vi "Begin.vi"() -> (0 "error out":errorcluster)   [LabVIEW 2013]
doc: "Called before other user functions, this VI is expected to open initial I/O refnums, load in file data, and do all program initialization. Notice that the <B>error out</B> terminal is simply used for data flow. Wiring it to other structures or subVIs ensures that this VI runs first."
uses:
  <vilib>/Rock Robotics/WPI/DriverStation/WPI_DriverStationRobotMode2.ctl
  <vilib>/Rock Robotics/WPI/Joystick/WPI_JoystickDeviceEnum.ctl
  <vilib>/Rock Robotics/SystemInterfaces/DIO/FPGA_DIOPWMChannel.ctl
  <vilib>/Rock Robotics/SystemInterfaces/Typedef/FPGA_TypedefDigitalModule.ctl
  <vilib>/Rock Robotics/SystemInterfaces/DIO/FPGA_DIOChannel.ctl
  <vilib>/Rock Robotics/SystemInterfaces/Typedef/FPGA_TypedefAnalogModuleForGyro.ctl
  <vilib>/Rock Robotics/SystemInterfaces/AI/FPGA_AIGyroChannel.ctl
  <vilib>/Rock Robotics/WPI/Solenoid/WPI_SolenoidChannel.ctl
  <vilib>/Rock Robotics/SystemInterfaces/AI/FPGA_AIChannel.ctl
  <vilib>/Rock Robotics/SystemInterfaces/DIO/FPGA_DIORelayChannel.ctl
  <vilib>/Rock Robotics/WPI/Relay/WPI_RelayDirection.ctl
  <vilib>/Rock Robotics/SystemInterfaces/Typedef/FPGA_TypedefSolenoidModule.ctl
  <vilib>/Rock Robotics/WPI/Solenoid/WPI_SolenoidValue.ctl
  <vilib>/Rock Robotics/WPI/SafetyOutput/WPI_SafetyOutputConfigMenu.ctl
  Robot Global Data.vi
  <vilib>/Rock Robotics/WPI/MotorControl/WPI_MotorControlOpen Talon.vi
  <vilib>/Rock Robotics/WPI/Counter/WPI_CounterDigitalInputToDigitalSource.vi
  <vilib>/Rock Robotics/WPI/Counter/WPI_CounterOpen Semi Period Mode.vi
  <vilib>/Rock Robotics/WPI/Solenoid/WPI_SolenoidOpenSingle.vi
  <vilib>/Rock Robotics/WPI/Solenoid/WPI_SolenoidOpenDouble.vi
  <vilib>/Rock Robotics/WPI/Solenoid/WPI_SolenoidSetEnum.vi
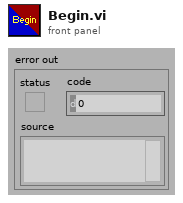
[diagram p1: front panel]
types:
  T1 = typedef "WPI_SafetyOutputConfigMenu.ctl" = enum16{"Enable", "Disable"}
  T2 = typedef "WPI_SolenoidValue.ctl" = enum16{"Off", "On", "Forward", "Reverse"}
  T3 = typedef "FPGA_AIChannel.ctl" = enum8{"AI 1", "AI 2", "AI 3", "AI 4", "AI 5", "AI 6", "AI 7", "AI 8", "Invalid"}
  T4 = typedef "WPI_SolenoidChannel.ctl" = enum8{"Solenoid 1", "Solenoid 2", "Solenoid 3", "Solenoid 4", "Solenoid 5", "Solenoid 6", "Solenoid 7", "Solenoid 8", "Invalid"}
  T5 = typedef "FPGA_TypedefSolenoidModule.ctl" = enum16{"Solenoid Module 1", "Solenoid Module 2"}
  T6 = typedef "WPI_RelayDirection.ctl" = enum16{"Both directions", "Forward only", "Reverse only"}
  T7 = typedef "FPGA_DIORelayChannel.ctl" = enum8{"Relay 1", "Relay 2", "Relay 3", "Relay 4", "Relay 5", "Relay 6", "Relay 7", "Relay 8", "Invalid"}
  T8 = typedef "FPGA_DIOPWMChannel.ctl" = enum8{"PWM 1", "PWM 2", "PWM 3", "PWM 4", "PWM 5", "PWM 6", "PWM 7", "PWM 8", "PWM 9", "PWM 10", "Invalid"}
  T9 = typedef "FPGA_TypedefDigitalModule.ctl" = enum16{"Digital Module 1", "Digital Module 2"}
  T10 = typedef "FPGA_DIOChannel.ctl" = enum8{"DIO 1", "DIO 2", "DIO 3", "DIO 4", "DIO 5", "DIO 6", "DIO 7", "DIO 8", "DIO 9", "DIO 10", "DIO 11", "DIO 12", "DIO 13", "DIO 14", "Invalid"}
  T11 = typedef "WPI_JoystickDeviceEnum.ctl" = enum16{"USB 1", "USB 2", "USB 3", "USB 4", "Kinect 1", "Kinect 2"}
  T12 = typedef "FPGA_AIGyroChannel.ctl" = enum8{"AI 1", "AI 2", "Invalid"}
  T13 = typedef "FPGA_TypedefAnalogModuleForGyro.ctl" = enum16{"Analog Module 1"}
  T14 = typedef "WPI_DriverStationRobotMode2.ctl" = enum16{"Autonomous Disabled", "Autonomous Enabled", "Teleop Disabled", "Teleop Enabled", "Timeout", "Finish", "Test Disabled", "Test Enabled"}
  T15 = typedef "WPI_SolenoidDevRef.ctl" = cluster{"DevStatus":errorcluster, "Solenoid Module":T5, "Forward Solenoid Channel":T4, "Reverse Solenoid Channel":T4}
  T16 = typedef "WPI_JoystickDevRef.ctl" = cluster{"Device":T11}
  T17 = typedef "WPI_AnalogChannelDevRef.ctl" = cluster{"DevStatus":errorcluster, "Analog Module":T18, "Analog Channel":T3}
  T18 = typedef "FPGA_TypedefAnalogModule.ctl" = enum16{"Analog Module 1", "Analog Module 2"}
  T19 = typedef "WPI_DigitalInputDevRef.ctl" = cluster{"DevStatus":errorcluster, "DIO Channel":T10, "Digital Module":T9}
  T20 = typedef "WPI_ServoDeviceRef.ctl" = cluster{"DeviceStatus":errorcluster, "Digital Module":T9, "PWM Channel":T8, "DeadBand":T21}
  T21 = typedef "WPI_PWMDeadband.ctl" = cluster{"Name":string, "maxPositivePwm":i32, "minPositivePwm":i32, "centerPwm":i32, "maxNegativePwm":i32, "minNegativePwm":i32, "angularRange":u16}
  T22 = typedef "FPGA_CounterEncoderSourceConvertionLVSourceType.ctl" = cluster{"DevStatus":errorcluster, "AnalogTriggerMode?":bool, "DigitalMode":cluster{"Digital Module":T9, "DIO Channel":T23}, "AnalogTriggerMode":cluster{"AnalogTriggerIndex":T24, "OutputType":T25}}
  T23 = typedef "FPGA_DIODigitalSourceChannel.ctl" = enum8{"DIO 1", "DIO 2", "DIO 3", "DIO 4", "DIO 5", "DIO 6", "DIO 7", "DIO 8", "DIO 9", "DIO 10", "DIO 11", "DIO 12", "DIO 13", "DIO 14", "Disabled"}
  T24 = typedef "FPGA_AnalogTriggerIndex.ctl" = enum8{"Trig 0", "Trig 1", "Trig 2", "Trig 3", "Trig 4", "Trig 5", "Trig 6", "Trig 7", "Invalid"}
  T25 = typedef "FPGA_AnalogTriggerOutType.ctl" = enum16{"InWindow", "TriggerState", "Rising", "Falling"}
  T26 = typedef "WPI_RelayDevRef.ctl" = cluster{"DevStatus":errorcluster, "Relay Channel":T7, "Digital Module":T9, "Relay Direction":T6}
  T27 = typedef "WPI_MotorControlDeviceRef.ctl" = cluster{"DeviceStatus":errorcluster, "Type":enum16{"PWM", "CAN"}, "PWM":cluster{"Digital Module":T9, "PWM Channel":T8, "DeadBand":T21}, "CAN":cluster{"Device Number":u8, "Control Mode":T28, "Semaphore":T29, "Max Vout":dbl}, "Invert":bool, "TransformRef":T30, "InvTransformRef":T30}
  T28 = typedef "WPI_CANJaguar_ControlMode.ctl" = enum8{"Percent VBus", "Current", "Speed", "Position", "Voltage"}
  T29 = typedef "Semaphore RefNum" = refnum<k1>
  T30 = typedef "WPI_PWMTransform_ConPane.ctl" = refnum<vi>
  T31 = typedef "WPI_GyroDevRef.ctl" = cluster{"DevStatus":errorcluster, "Analog Module":T18, "Analog Channel":T3, "Offset":dbl, "Gain (VoltsPerDegree/Second)":dbl}
  T32 = typedef "WPI_CounterDevRef.ctl" = cluster{"DevStatus":errorcluster, "CntIndex":T33}
  T33 = typedef "FPGA_CounterCtrSystemIndex.ctl" = enum8{"Ctr 0", "Ctr 1", "Ctr 2", "Ctr 3", "Ctr 4", "Ctr 5", "Ctr 6", "Ctr 7", "Invalid"}
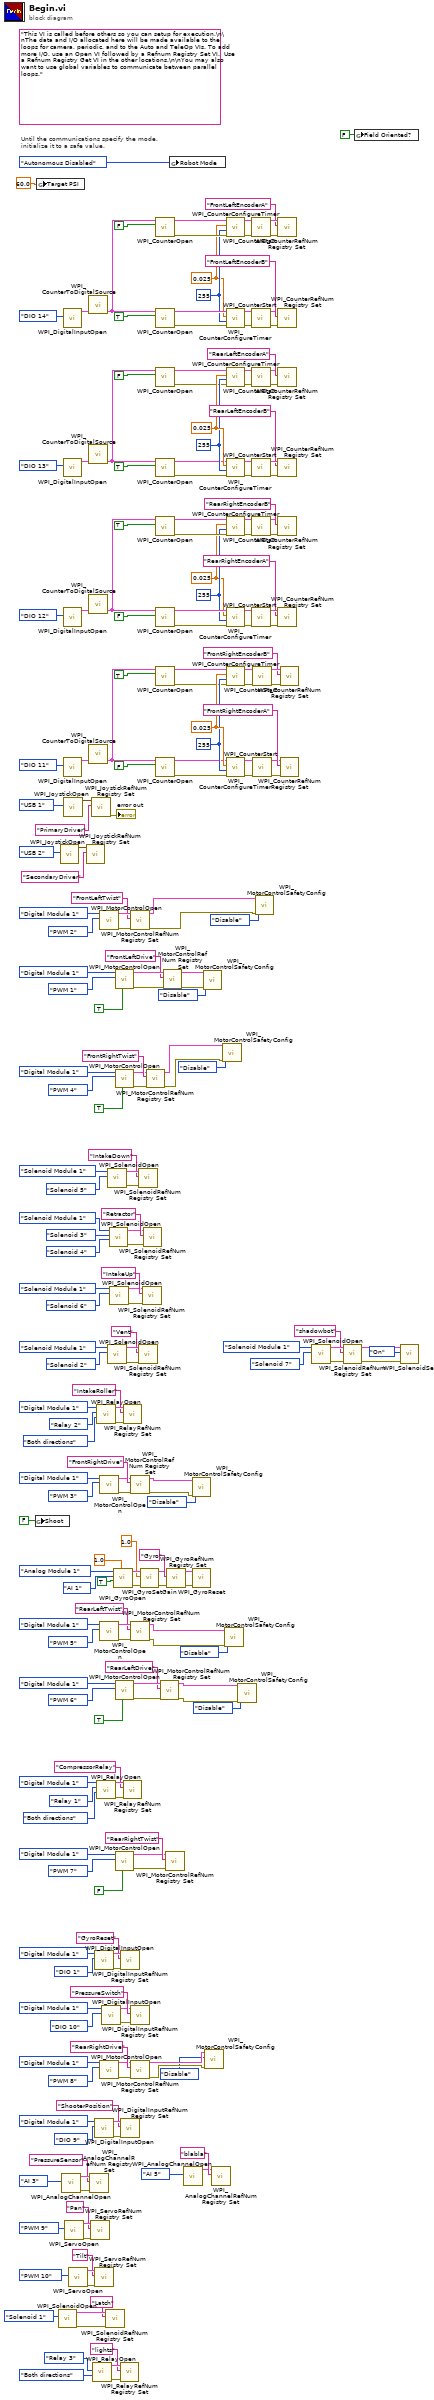
[diagram p0: block diagram]
diagram:
  w145 = 0.025 ("MaxPeriod (sec)")
  w144 = u8 255 ("Number Samples to Average")
  w146 = 0.025 ("MaxPeriod (sec)")
  w147 = u8 255 ("Number Samples to Average")
  w185 = 0.025 ("MaxPeriod (sec)")
  w184 = u8 255 ("Number Samples to Average")
  w187 = 0.025 ("MaxPeriod (sec)")
  w188 = u8 255 ("Number Samples to Average")
  (unwired) "This VI is called before others so you can setup for execution.\n\nThe data and I/O allocated here will be made available to the loops for camera, periodic, and to the Auto and TeleOp VIs. To add more I/O, use an Open VI followed by a Refnum Registry Set VI.  Use a Refnum Registry Get VI in the other locations.\n\nYou may also want to use global variables to communicate between parallel loops."
  # "Until the communications specify the mode,\ninitialize it to a safe value."
  n1 = global write "Robot Global Data.vi" "Shoot"(FALSE ("Shoot")) -> ()
  n2 = global write "Robot Global Data.vi" "Target PSI"(60.0 ("Target PSI")) -> ()
  n3 = call-poly <vilib>:"WPI_SolenoidOpen.vi"("Solenoid Channel"=WPI_SolenoidChannel."Solenoid 1") -> ("error out"=w34:errorcluster, "SolenoidDevRef"=w35:T15)  [unwired: 9 in]
  n4 = call <vilib>:"WPI_JoystickOpen.vi"("JoystickDevice"=WPI_JoystickDeviceEnum."USB 2") -> ("JoystickDevRef"=w108:T16)  [unwired: 10 in]
  n5 = call <vilib>:"WPI_AnalogChannelOpen.vi"("Analog Channel"=FPGA_AIChannel."AI 3") -> ("error out"=w89:errorcluster, "AIDeviceRef"=w88:T17)  [unwired: 9 in]
  n6 = call <vilib>:"WPI_DigitalInputOpen.vi"("DIO Channel"=FPGA_DIOChannel."DIO 14") -> ("DigitalInputDevRef"=w202:T19)  [unwired: 9 in, 1 out]
  n7 = call <vilib>:"WPI_DigitalInputOpen.vi"("DIO Channel"=FPGA_DIOChannel."DIO 13") -> ("DigitalInputDevRef"=w130:T19)  [unwired: 9 in, 1 out]
  n8 = call <vilib>:"WPI_DigitalInputOpen.vi"("DIO Channel"=FPGA_DIOChannel."DIO 12") -> ("DigitalInputDevRef"=w163:T19)  [unwired: 9 in, 1 out]
  n9 = call <vilib>:"WPI_DigitalInputOpen.vi"("DIO Channel"=FPGA_DIOChannel."DIO 11") -> ("DigitalInputDevRef"=w168:T19)  [unwired: 9 in, 1 out]
  n10 = call <vilib>:"WPI_JoystickOpen.vi"("JoystickDevice"=WPI_JoystickDeviceEnum."USB 1") -> ("JoystickDevRef"=w250:T16)  [unwired: 10 in]
  n11 = call <vilib>:"WPI_ServoOpen.vi"("PWM Channel"=FPGA_DIOPWMChannel."PWM 9") -> ("error out"=w50:errorcluster, "ServoDeviceRef"=w49:T20)  [unwired: 9 in]
  n12 = call <vilib>:"WPI_ServoOpen.vi"("PWM Channel"=FPGA_DIOPWMChannel."PWM 10") -> ("error out"=w48:errorcluster, "ServoDeviceRef"=w47:T20)  [unwired: 9 in]
  n13 = call <vilib>:"WPI_JoystickRefNum Registry Set.vi"("refnum name"="SecondaryDriver", "JoystickDevRef"=w108) -> ()  [unwired: 8 in, 2 out]
  n14 = call-poly <vilib>:"WPI_CounterToDigitalSource.vi"("DigitalInputDevRef"=w202) -> ("Digital Source"=w186:T22)  [unwired: 6 in]
  n15 = call-poly <vilib>:"WPI_CounterToDigitalSource.vi"("DigitalInputDevRef"=w130) -> ("Digital Source"=w125:T22)  [unwired: 6 in]
  n16 = call-poly <vilib>:"WPI_CounterToDigitalSource.vi"("DigitalInputDevRef"=w163) -> ("Digital Source"=w124:T22)  [unwired: 6 in]
  n17 = call-poly <vilib>:"WPI_CounterToDigitalSource.vi"("DigitalInputDevRef"=w168) -> ("Digital Source"=w123:T22)  [unwired: 6 in]
  n18 = call <vilib>:"WPI_AnalogChannelRefNum Registry Set.vi"("error in (no error)"=w89, "refnum name"="PressureSensor", "AIDeviceRef"=w88) -> ()  [unwired: 7 in, 2 out]
  n19 = call <vilib>:"WPI_ServoRefNum Registry Set.vi"("error in (no error)"=w50, "refnum name"="Pan", "ServoDeviceRef"=w49) -> ()  [unwired: 7 in, 2 out]
  n20 = call <vilib>:"WPI_JoystickRefNum Registry Set.vi"("refnum name"="PrimaryDriver", "JoystickDevRef"=w250) -> ("error out"=→"error out":errorcluster)  [unwired: 8 in, 1 out]
  n21 = call <vilib>:"WPI_RelayOpen.vi"("Relay Direction"=WPI_RelayDirection."Both directions", "Relay Channel"=FPGA_DIORelayChannel."Relay 3") -> ("error out"=w40:errorcluster, "RelayDevRef"=w39:T26)  [unwired: 8 in]
  n22 = call <vilib>:"WPI_DigitalInputOpen.vi"("DIO Channel"=FPGA_DIOChannel."DIO 1", "Digital Module (Module 1)"=FPGA_TypedefDigitalModule."Digital Module 1") -> ("error out"=w71:errorcluster, "DigitalInputDevRef"=w70:T19)  [unwired: 8 in]
  n23 = call <vilib>:"WPI_DigitalInputOpen.vi"("DIO Channel"=FPGA_DIOChannel."DIO 9", "Digital Module (Module 1)"=FPGA_TypedefDigitalModule."Digital Module 1") -> ("error out"=w106:errorcluster, "DigitalInputDevRef"=w105:T19)  [unwired: 8 in]
  n24 = call <vilib>:"WPI_ServoRefNum Registry Set.vi"("error in (no error)"=w48, "refnum name"="Tilt", "ServoDeviceRef"=w47) -> ()  [unwired: 7 in, 2 out]
  n25 = call <vilib>:"WPI_RelayOpen.vi"("Relay Direction"=WPI_RelayDirection."Both directions", "Relay Channel"=FPGA_DIORelayChannel."Relay 2", "Digital Module (Module 1)"=FPGA_TypedefDigitalModule."Digital Module 1") -> ("error out"=w53:errorcluster, "RelayDevRef"=w52:T26)  [unwired: 7 in]
  n26 = call <vilib>:"WPI_RelayOpen.vi"("Relay Direction"=WPI_RelayDirection."Both directions", "Relay Channel"=FPGA_DIORelayChannel."Relay 1", "Digital Module (Module 1)"=FPGA_TypedefDigitalModule."Digital Module 1") -> ("error out"=w82:errorcluster, "RelayDevRef"=w81:T26)  [unwired: 7 in]
  n27 = call-poly <vilib>:"WPI_MotorControlOpen.vi"("PWM Channel"=FPGA_DIOPWMChannel."PWM 2", "Digital Module (Module 1)"=FPGA_TypedefDigitalModule."Digital Module 1") -> ("error out"=w248:errorcluster, "MotorControlDeviceRef"=w247:T27)  [unwired: 8 in]
  n28 = call-poly <vilib>:"WPI_MotorControlOpen.vi"("PWM Channel"=FPGA_DIOPWMChannel."PWM 3", "Digital Module (Module 1)"=FPGA_TypedefDigitalModule."Digital Module 1") -> ("error out"=w234:errorcluster, "MotorControlDeviceRef"=w235:T27)  [unwired: 8 in]
  n29 = call-poly <vilib>:"WPI_MotorControlOpen.vi"("PWM Channel"=FPGA_DIOPWMChannel."PWM 5", "Digital Module (Module 1)"=FPGA_TypedefDigitalModule."Digital Module 1") -> ("error out"=w228:errorcluster, "MotorControlDeviceRef"=w227:T27)  [unwired: 8 in]
  n30 = call-poly <vilib>:"WPI_MotorControlOpen.vi"("PWM Channel"=FPGA_DIOPWMChannel."PWM 8", "Digital Module (Module 1)"=FPGA_TypedefDigitalModule."Digital Module 1") -> ("error out"=w214:errorcluster, "MotorControlDeviceRef"=w215:T27)  [unwired: 8 in]
  n31 = call <vilib>:"WPI_DigitalInputOpen.vi"("DIO Channel"=FPGA_DIOChannel."DIO 10", "Digital Module (Module 1)"=FPGA_TypedefDigitalModule."Digital Module 1") -> ("error out"=w72:errorcluster, "DigitalInputDevRef"=w73:T19)  [unwired: 8 in]
  n32 = call <vilib>:"WPI_SolenoidRefNum Registry Set.vi"("error in (no error)"=w34, "refnum name"="Latch", "SolenoidDevRef"=w35) -> ()  [unwired: 7 in, 2 out]
  n33 = call-poly <vilib>:"WPI_SolenoidOpen.vi"("Solenoid Channel"=WPI_SolenoidChannel."Solenoid 5" ("Forward Solenoid Channel"), "Solenoid Module (Module 1)"=FPGA_TypedefSolenoidModule."Solenoid Module 1") -> ("error out"=w63:errorcluster, "SolenoidDevRef"=w64:T15)  [unwired: 8 in]
  n34 = call-poly <vilib>:"WPI_SolenoidOpen.vi"("Solenoid Channel"=WPI_SolenoidChannel."Solenoid 2" ("Forward Solenoid Channel"), "Solenoid Module (Module 1)"=FPGA_TypedefSolenoidModule."Solenoid Module 1") -> ("error out"=w96:errorcluster, "SolenoidDevRef"=w95:T15)  [unwired: 8 in]
  n35 = call-poly <vilib>:"WPI_SolenoidOpen.vi"("Reverse Solenoid Channel"=WPI_SolenoidChannel."Solenoid 4", "Forward Solenoid Channel"=WPI_SolenoidChannel."Solenoid 3", "Solenoid Module (Module 1)"=FPGA_TypedefSolenoidModule."Solenoid Module 1") -> ("error out"=w97:errorcluster, "SolenoidDevRef"=w98:T15)  [unwired: 7 in]
  n36 = call-poly <vilib>:"WPI_SolenoidOpen.vi"("Solenoid Channel"=WPI_SolenoidChannel."Solenoid 6" ("Forward Solenoid Channel"), "Solenoid Module (Module 1)"=FPGA_TypedefSolenoidModule."Solenoid Module 1") -> ("error out"=w60:errorcluster, "SolenoidDevRef"=w59:T15)  [unwired: 8 in]
  n37 = call <vilib>:"WPI_GyroOpen.vi"("Calibration Time (s)"=1.0, "Calibrate On Open"=TRUE, "Analog Channel"=FPGA_AIGyroChannel."AI 1", "Analog Module (Module 1)"=FPGA_TypedefAnalogModuleForGyro."Analog Module 1") -> ("error out"=w110:errorcluster, "GyroDevRef"=w113:T31)  [unwired: 5 in, 1 out]
  n38 = call-poly <vilib>:"WPI_MotorControlOpen.vi"("Invert"=TRUE, "PWM Channel"=FPGA_DIOPWMChannel."PWM 1", "Digital Module (Module 1)"=FPGA_TypedefDigitalModule."Digital Module 1") -> ("error out"=w243:errorcluster, "MotorControlDeviceRef"=w242:T27)  [unwired: 7 in]
  n39 = call-poly <vilib>:"WPI_MotorControlOpen.vi"("Invert"=TRUE, "PWM Channel"=FPGA_DIOPWMChannel."PWM 4", "Digital Module (Module 1)"=FPGA_TypedefDigitalModule."Digital Module 1") -> ("error out"=w229:errorcluster, "MotorControlDeviceRef"=w230:T27)  [unwired: 7 in]
  n40 = call-poly <vilib>:"WPI_MotorControlOpen.vi"("Invert"=TRUE, "PWM Channel"=FPGA_DIOPWMChannel."PWM 6", "Digital Module (Module 1)"=FPGA_TypedefDigitalModule."Digital Module 1") -> ("error out"=w223:errorcluster, "MotorControlDeviceRef"=w222:T27)  [unwired: 7 in]
  n41 = call-poly <vilib>:"WPI_MotorControlOpen.vi"("Invert"=FALSE, "PWM Channel"=FPGA_DIOPWMChannel."PWM 7", "Digital Module (Module 1)"=FPGA_TypedefDigitalModule."Digital Module 1") -> ("error out"=w209:errorcluster, "MotorControlDeviceRef"=w210:T27)  [unwired: 7 in]
  n42 = call <vilib>:"WPI_RelayRefNum Registry Set.vi"("error in (no error)"=w40, "refnum name"="lights", "RelayDevRef"=w39) -> ()  [unwired: 7 in, 2 out]
  n43 = call <vilib>:"WPI_DigitalInputRefNum Registry Set.vi"("error in (no error)"=w71, "refnum name"="GyroReset", "DigitalInputDevRef"=w70) -> ()  [unwired: 7 in, 2 out]
  n44 = call <vilib>:"WPI_DigitalInputRefNum Registry Set.vi"("error in (no error)"=w106, "refnum name"="ShooterPosition", "DigitalInputDevRef"=w105) -> ()  [unwired: 7 in, 2 out]
  n45 = call <vilib>:"WPI_RelayRefNum Registry Set.vi"("error in (no error)"=w53, "refnum name"="IntakeRoller", "RelayDevRef"=w52) -> ()  [unwired: 7 in, 2 out]
  n46 = call <vilib>:"WPI_RelayRefNum Registry Set.vi"("error in (no error)"=w82, "refnum name"="CompressorRelay", "RelayDevRef"=w81) -> ()  [unwired: 7 in, 2 out]
  n47 = call <vilib>:"WPI_MotorControlRefNum Registry Set.vi"("error in (no error)"=w248, "refnum name"="FrontLeftTwist", "MotorControlDevRef"=w247) -> ("error out"=w10:errorcluster, "MotorControlDevRef"=w11:T27)  [unwired: 7 in]
  n48 = call <vilib>:"WPI_MotorControlRefNum Registry Set.vi"("error in (no error)"=w234, "refnum name"="FrontRightDrive", "MotorControlDevRef"=w235) -> ("error out"=w16:errorcluster, "MotorControlDevRef"=w17:T27)  [unwired: 7 in]
  n49 = call <vilib>:"WPI_MotorControlRefNum Registry Set.vi"("error in (no error)"=w228, "refnum name"="RearLeftTwist", "MotorControlDevRef"=w227) -> ("error out"=w4:errorcluster, "MotorControlDevRef"=w5:T27)  [unwired: 7 in]
  n50 = call <vilib>:"WPI_DigitalInputRefNum Registry Set.vi"("error in (no error)"=w72, "refnum name"="PressureSwitch", "DigitalInputDevRef"=w73) -> ()  [unwired: 7 in, 2 out]
  n51 = call <vilib>:"WPI_MotorControlRefNum Registry Set.vi"("error in (no error)"=w214, "refnum name"="RearRightDrive", "MotorControlDevRef"=w215) -> ("error out"=w14:errorcluster, "MotorControlDevRef"=w15:T27)  [unwired: 7 in]
  n52 = call <vilib>:"WPI_SolenoidRefNum Registry Set.vi"("error in (no error)"=w63, "refnum name"="IntakeDown", "SolenoidDevRef"=w64) -> ()  [unwired: 7 in, 2 out]
  n53 = call <vilib>:"WPI_SolenoidRefNum Registry Set.vi"("error in (no error)"=w96, "refnum name"="Vent", "SolenoidDevRef"=w95) -> ()  [unwired: 7 in, 2 out]
  n54 = call <vilib>:"WPI_GyroSetGain.vi"("error in (no error)"=w110, "Gain (VoltsPerDegree/Second)"=1.0, "GyroDevRef"=w113) -> ("error out"=w111:errorcluster, "GyroDevRef"=w112:T31)  [unwired: 7 in]
  n55 = call <vilib>:"WPI_SolenoidRefNum Registry Set.vi"("error in (no error)"=w60, "refnum name"="IntakeUp", "SolenoidDevRef"=w59) -> ()  [unwired: 7 in, 2 out]
  n56 = call <vilib>:"WPI_SolenoidRefNum Registry Set.vi"("error in (no error)"=w97, "refnum name"="Retractor", "SolenoidDevRef"=w98) -> ()  [unwired: 7 in, 2 out]
  n57 = call <vilib>:"WPI_MotorControlRefNum Registry Set.vi"("error in (no error)"=w229, "refnum name"="FrontRightTwist", "MotorControlDevRef"=w230) -> ("error out"=w7:errorcluster, "MotorControlDevRef"=w8:T27)  [unwired: 7 in]
  n58 = call-poly <vilib>:"WPI_CounterOpen.vi"("High Pulse (T)"=FALSE, "Source"=w186) -> ("error out"=w196:errorcluster, "CounterDevRef"=w195:T32)  [unwired: 8 in]
  n59 = call-poly <vilib>:"WPI_CounterOpen.vi"("High Pulse (T)"=TRUE, "Source"=w186) -> ("error out"=w192:errorcluster, "CounterDevRef"=w191:T32)  [unwired: 8 in]
  n60 = call-poly <vilib>:"WPI_CounterOpen.vi"("High Pulse (T)"=FALSE, "Source"=w125) -> ("error out"=w136:errorcluster, "CounterDevRef"=w137:T32)  [unwired: 8 in]
  n61 = call-poly <vilib>:"WPI_CounterOpen.vi"("High Pulse (T)"=TRUE, "Source"=w125) -> ("error out"=w140:errorcluster, "CounterDevRef"=w141:T32)  [unwired: 8 in]
  n62 = call-poly <vilib>:"WPI_CounterOpen.vi"("High Pulse (T)"=TRUE, "Source"=w124) -> ("error out"=w151:errorcluster, "CounterDevRef"=w150:T32)  [unwired: 8 in]
  n63 = call-poly <vilib>:"WPI_CounterOpen.vi"("High Pulse (T)"=FALSE, "Source"=w124) -> ("error out"=w155:errorcluster, "CounterDevRef"=w154:T32)  [unwired: 8 in]
  n64 = call-poly <vilib>:"WPI_CounterOpen.vi"("High Pulse (T)"=TRUE, "Source"=w123) -> ("error out"=w180:errorcluster, "CounterDevRef"=w181:T32)  [unwired: 8 in]
  n65 = call-poly <vilib>:"WPI_CounterOpen.vi"("High Pulse (T)"=FALSE, "Source"=w123) -> ("error out"=w176:errorcluster, "CounterDevRef"=w177:T32)  [unwired: 8 in]
  n66 = call <vilib>:"WPI_MotorControlRefNum Registry Set.vi"("error in (no error)"=w223, "refnum name"="RearLeftDrive", "MotorControlDevRef"=w222) -> ("error out"=w1:errorcluster, "MotorControlDevRef"=w2:T27)  [unwired: 7 in]
  n67 = call <vilib>:"WPI_MotorControlRefNum Registry Set.vi"("error in (no error)"=w243, "refnum name"="FrontLeftDrive", "MotorControlDevRef"=w242) -> ("error out"=w20:errorcluster, "MotorControlDevRef"=w21:T27)  [unwired: 7 in]
  n68 = call <vilib>:"WPI_MotorControlRefNum Registry Set.vi"("error in (no error)"=w209, "refnum name"="RearRightTwist", "MotorControlDevRef"=w210) -> ()  [unwired: 7 in, 2 out]
  n69 = call <vilib>:"WPI_GyroRefNum Registry Set.vi"("error in (no error)"=w111, "refnum name"="Gyro", "GyroDevRef"=w112) -> ("error out"=w84:errorcluster, "GyroDevRef"=w83:T31)  [unwired: 7 in]
  n70 = global write "Robot Global Data.vi" "Robot Mode"(WPI_DriverStationRobotMode2."Autonomous Disabled" ("Robot Mode")) -> ()
  n71 = call <vilib>:"WPI_AnalogChannelOpen.vi"("Analog Channel"=FPGA_AIChannel."AI 5") -> ("AIDeviceRef"=w25:T17)  [unwired: 9 in, 1 out]
  n72 = call <vilib>:"WPI_MotorControlSafetyConfig.vi"("error in (no error)"=w16, "mode"=WPI_SafetyOutputConfigMenu."Disable", "MotorControlDevRef"=w17) -> ()  [unwired: 7 in, 2 out]
  n73 = call <vilib>:"WPI_GyroReset.vi"("error in (no error)"=w84, "GyroDevRef"=w83) -> ()  [unwired: 8 in, 2 out]
  n74 = call <vilib>:"WPI_MotorControlSafetyConfig.vi"("error in (no error)"=w20, "mode"=WPI_SafetyOutputConfigMenu."Disable", "MotorControlDevRef"=w21) -> ()  [unwired: 7 in, 2 out]
  n75 = call <vilib>:"WPI_MotorControlSafetyConfig.vi"("error in (no error)"=w14, "mode"=WPI_SafetyOutputConfigMenu."Disable", "MotorControlDevRef"=w15) -> ()  [unwired: 7 in, 2 out]
  n76 = call <vilib>:"WPI_AnalogChannelRefNum Registry Set.vi"("refnum name"="blabla", "AIDeviceRef"=w25) -> ()  [unwired: 8 in, 2 out]
  n77 = call <vilib>:"WPI_MotorControlSafetyConfig.vi"("error in (no error)"=w7, "mode"=WPI_SafetyOutputConfigMenu."Disable", "MotorControlDevRef"=w8) -> ()  [unwired: 7 in, 2 out]
  n78 = call <vilib>:"WPI_MotorControlSafetyConfig.vi"("error in (no error)"=w4, "mode"=WPI_SafetyOutputConfigMenu."Disable", "MotorControlDevRef"=w5) -> ()  [unwired: 7 in, 2 out]
  n79 = call <vilib>:"WPI_CounterConfigureTimer.vi"("error in (no error)"=w196, "Number Samples to Average"=w188, "MaxPeriod (sec)"=w187, "CounterDevRef in"=w195) -> ("error out"=w193:errorcluster, "CounterDevRef out"=w194:T32)  [unwired: 6 in]
  n80 = call <vilib>:"WPI_CounterConfigureTimer.vi"("error in (no error)"=w192, "Number Samples to Average"=w188, "MaxPeriod (sec)"=w187, "CounterDevRef in"=w191) -> ("error out"=w189:errorcluster, "CounterDevRef out"=w190:T32)  [unwired: 6 in]
  n81 = call <vilib>:"WPI_CounterConfigureTimer.vi"("error in (no error)"=w136, "Number Samples to Average"=w144, "MaxPeriod (sec)"=w145, "CounterDevRef in"=w137) -> ("error out"=w139:errorcluster, "CounterDevRef out"=w138:T32)  [unwired: 6 in]
  n82 = call <vilib>:"WPI_CounterConfigureTimer.vi"("error in (no error)"=w140, "Number Samples to Average"=w144, "MaxPeriod (sec)"=w145, "CounterDevRef in"=w141) -> ("error out"=w143:errorcluster, "CounterDevRef out"=w142:T32)  [unwired: 6 in]
  n83 = call <vilib>:"WPI_CounterConfigureTimer.vi"("error in (no error)"=w151, "Number Samples to Average"=w147, "MaxPeriod (sec)"=w146, "CounterDevRef in"=w150) -> ("error out"=w148:errorcluster, "CounterDevRef out"=w149:T32)  [unwired: 6 in]
  n84 = call <vilib>:"WPI_CounterConfigureTimer.vi"("error in (no error)"=w155, "Number Samples to Average"=w147, "MaxPeriod (sec)"=w146, "CounterDevRef in"=w154) -> ("error out"=w152:errorcluster, "CounterDevRef out"=w153:T32)  [unwired: 6 in]
  n85 = call <vilib>:"WPI_CounterConfigureTimer.vi"("error in (no error)"=w180, "Number Samples to Average"=w184, "MaxPeriod (sec)"=w185, "CounterDevRef in"=w181) -> ("error out"=w183:errorcluster, "CounterDevRef out"=w182:T32)  [unwired: 6 in]
  n86 = call <vilib>:"WPI_CounterConfigureTimer.vi"("error in (no error)"=w176, "Number Samples to Average"=w184, "MaxPeriod (sec)"=w185, "CounterDevRef in"=w177) -> ("error out"=w179:errorcluster, "CounterDevRef out"=w178:T32)  [unwired: 6 in]
  n87 = call <vilib>:"WPI_MotorControlSafetyConfig.vi"("error in (no error)"=w1, "mode"=WPI_SafetyOutputConfigMenu."Disable", "MotorControlDevRef"=w2) -> ()  [unwired: 7 in, 2 out]
  n88 = call <vilib>:"WPI_CounterStart.vi"("error in (no error)"=w193, "CounterDevRef in"=w194) -> ("error out"=w206:errorcluster, "CounterDevRef out"=w205:T32)  [unwired: 8 in]
  n89 = call <vilib>:"WPI_CounterStart.vi"("error in (no error)"=w189, "CounterDevRef in"=w190) -> ("error out"=w200:errorcluster, "CounterDevRef out"=w201:T32)  [unwired: 8 in]
  n90 = call <vilib>:"WPI_CounterStart.vi"("error in (no error)"=w139, "CounterDevRef in"=w138) -> ("error out"=w126:errorcluster, "CounterDevRef out"=w127:T32)  [unwired: 8 in]
  n91 = call <vilib>:"WPI_CounterStart.vi"("error in (no error)"=w143, "CounterDevRef in"=w142) -> ("error out"=w132:errorcluster, "CounterDevRef out"=w131:T32)  [unwired: 8 in]
  n92 = call <vilib>:"WPI_CounterStart.vi"("error in (no error)"=w148, "CounterDevRef in"=w149) -> ("error out"=w159:errorcluster, "CounterDevRef out"=w160:T32)  [unwired: 8 in]
  n93 = call <vilib>:"WPI_CounterStart.vi"("error in (no error)"=w152, "CounterDevRef in"=w153) -> ("error out"=w165:errorcluster, "CounterDevRef out"=w164:T32)  [unwired: 8 in]
  n94 = call <vilib>:"WPI_CounterStart.vi"("error in (no error)"=w183, "CounterDevRef in"=w182) -> ("error out"=w172:errorcluster, "CounterDevRef out"=w171:T32)  [unwired: 8 in]
  n95 = call <vilib>:"WPI_CounterStart.vi"("error in (no error)"=w179, "CounterDevRef in"=w178) -> ("error out"=w166:errorcluster, "CounterDevRef out"=w167:T32)  [unwired: 8 in]
  n96 = call <vilib>:"WPI_MotorControlSafetyConfig.vi"("error in (no error)"=w10, "mode"=WPI_SafetyOutputConfigMenu."Disable", "MotorControlDevRef"=w11) -> ()  [unwired: 7 in, 2 out]
  n97 = call <vilib>:"WPI_CounterRefNum Registry Set.vi"("error in (no error)"=w206, "refnum name"="FrontLeftEncoderA", "CounterDevRef"=w205) -> ()  [unwired: 7 in, 2 out]
  n98 = call <vilib>:"WPI_CounterRefNum Registry Set.vi"("error in (no error)"=w200, "refnum name"="FrontLeftEncoderB", "CounterDevRef"=w201) -> ()  [unwired: 7 in, 2 out]
  n99 = call <vilib>:"WPI_CounterRefNum Registry Set.vi"("error in (no error)"=w126, "refnum name"="RearLeftEncoderA", "CounterDevRef"=w127) -> ()  [unwired: 7 in, 2 out]
  n100 = call <vilib>:"WPI_CounterRefNum Registry Set.vi"("error in (no error)"=w132, "refnum name"="RearLeftEncoderB", "CounterDevRef"=w131) -> ()  [unwired: 7 in, 2 out]
  n101 = call <vilib>:"WPI_CounterRefNum Registry Set.vi"("error in (no error)"=w159, "refnum name"="RearRightEncoderB", "CounterDevRef"=w160) -> ()  [unwired: 7 in, 2 out]
  n102 = call <vilib>:"WPI_CounterRefNum Registry Set.vi"("error in (no error)"=w165, "refnum name"="RearRightEncoderA", "CounterDevRef"=w164) -> ()  [unwired: 7 in, 2 out]
  n103 = call <vilib>:"WPI_CounterRefNum Registry Set.vi"("error in (no error)"=w172, "refnum name"="FrontRightEncoderB", "CounterDevRef"=w171) -> ()  [unwired: 7 in, 2 out]
  n104 = call <vilib>:"WPI_CounterRefNum Registry Set.vi"("error in (no error)"=w166, "refnum name"="FrontRightEncoderA", "CounterDevRef"=w167) -> ()  [unwired: 7 in, 2 out]
  n105 = call-poly <vilib>:"WPI_SolenoidOpen.vi"("Solenoid Channel"=WPI_SolenoidChannel."Solenoid 7" ("Forward Solenoid Channel"), "Solenoid Module (Module 1)"=FPGA_TypedefSolenoidModule."Solenoid Module 1") -> ("error out"=w32:errorcluster, "SolenoidDevRef"=w31:T15)  [unwired: 8 in]
  n106 = call <vilib>:"WPI_SolenoidRefNum Registry Set.vi"("error in (no error)"=w32, "refnum name"="shadowbot", "SolenoidDevRef"=w31) -> ("error out"=w23:errorcluster, "SolenoidDevRef"=w24:T15)  [unwired: 7 in]
  n107 = global write "Robot Global Data.vi" "Field Oriented?"(FALSE ("Field Oriented?")) -> ()
  n108 = call-poly <vilib>:"WPI_SolenoidSet.vi"("error in (no error)"=w23, "Value"=WPI_SolenoidValue."On", "SolenoidDevRef"=w24) -> ()  [unwired: 7 in, 2 out]
